vi "Setup for ISTR.vi"(7 "String":u8, 8 "error in (no error)":errorcluster, 9 "Position in":u32, 10 "Cree Comms in":refnum<class "Cree Communications.lvclass">, 11 "Calibration in":refnum<class "Calibration.lvclass">) -> (0 "error out":errorcluster, 1 "Position out":u32, 2 "Cree Comms out":refnum<class "Cree Communications.lvclass">, 3 "Calibration out":refnum<class "Calibration.lvclass">)   [LabVIEW 2015, in "Calibration.lvclass"]
doc: "Turns off the strings not being calibrated. Sets Dim command to 100."
uses:
  Calibration.lvclass
  Classes/Cree Communications/Class/Cree Communications.lvclass
  Classes/Cree Communications/Cree Comms Messages/Write Dim Level/Set Dim Level.lvclass
  Classes/Cree Communications/Cree Comms Messages/CC Message/CC Message.lvclass/CC Message.ctl
  Classes/Cree Communications/Cree Comms Messages/Set Current Reference/Set String Current Ref.lvclass
  Classes/Cree Communications/Cree Comms Messages/CC Message/CC Message.lvclass
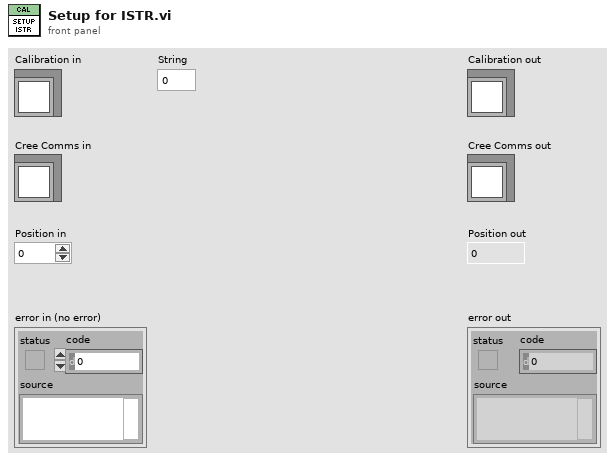
[diagram p1: front panel]
types:
  T1 = cluster{"Current Reference":dbl, "String":enum16{"Red", "BSY1", "BSY2"}}
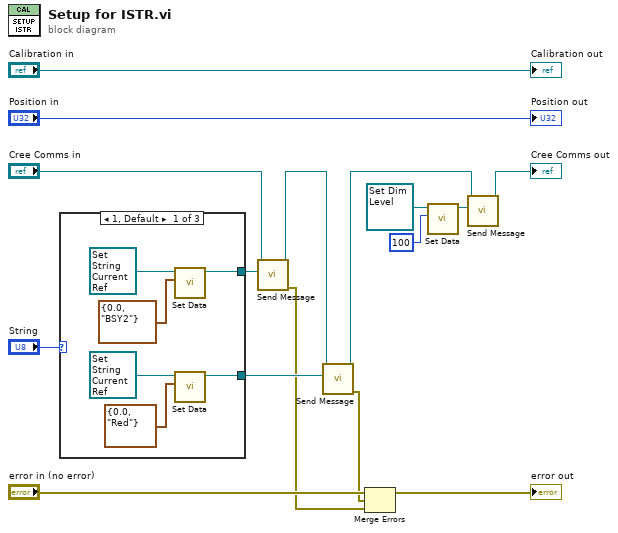
[diagram p0: block diagram]
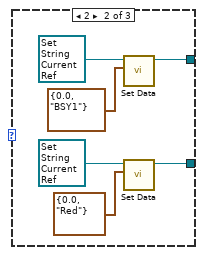
[diagram p2: hidden frame]
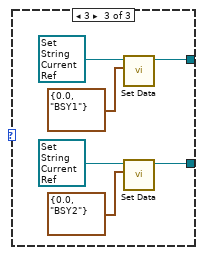
[diagram p3: hidden frame]
diagram:
  n1 = case shown="1, Default" "String" {
    tunnel: [w18 w24 w30] -> w10
    tunnel: [w17 w23 w29] -> w9
    frame 1, Default {
      n2 = call "Set Data.vi"("Data"=T1 {"Current Reference"=0.0, "String"=enum."BSY2"} ("Message Type"), "CC Message in"=refnum<class "Set String Current Ref.lvclass"> refnum ("Cree Comms Messages.lvlib:Set String Current Ref.lvclass")) -> ("CC Message out"=w18:refnum<class "Set String Current Ref.lvclass">)  [unwired: 8 in, 1 out]
      n3 = call "Set Data.vi"("Data"=T1 {"Current Reference"=0.0, "String"=enum."Red"} ("Message Type"), "CC Message in"=refnum<class "Set String Current Ref.lvclass"> refnum ("Cree Comms Messages.lvlib:Set String Current Ref.lvclass")) -> ("CC Message out"=w17:refnum<class "Set String Current Ref.lvclass">)  [unwired: 8 in, 1 out]
    }
    frame 2 {
      n4 = call "Set Data.vi"("Data"=T1 {"Current Reference"=0.0, "String"=enum."BSY1"} ("Message Type"), "CC Message in"=refnum<class "Set String Current Ref.lvclass"> refnum ("Cree Comms Messages.lvlib:Set String Current Ref.lvclass")) -> ("CC Message out"=w24:refnum<class "Set String Current Ref.lvclass">)  [unwired: 8 in, 1 out]
      n5 = call "Set Data.vi"("Data"=T1 {"Current Reference"=0.0, "String"=enum."Red"} ("Message Type"), "CC Message in"=refnum<class "Set String Current Ref.lvclass"> refnum ("Cree Comms Messages.lvlib:Set String Current Ref.lvclass")) -> ("CC Message out"=w23:refnum<class "Set String Current Ref.lvclass">)  [unwired: 8 in, 1 out]
    }
    frame 3 {
      n6 = call "Set Data.vi"("Data"=T1 {"Current Reference"=0.0, "String"=enum."BSY1"} ("Message Type"), "CC Message in"=refnum<class "Set String Current Ref.lvclass"> refnum ("Cree Comms Messages.lvlib:Set String Current Ref.lvclass")) -> ("CC Message out"=w30:refnum<class "Set String Current Ref.lvclass">)  [unwired: 8 in, 1 out]
      n7 = call "Set Data.vi"("Data"=T1 {"Current Reference"=0.0, "String"=enum."BSY2"} ("Message Type"), "CC Message in"=refnum<class "Set String Current Ref.lvclass"> refnum ("Cree Comms Messages.lvlib:Set String Current Ref.lvclass")) -> ("CC Message out"=w29:refnum<class "Set String Current Ref.lvclass">)  [unwired: 8 in, 1 out]
    }
  }
  n8 = call "Send Message.vi"("Cree Comms Message"=w10, "Acrobat Template in"="Cree Comms in") -> ("error out"=w6:errorcluster, "Acrobat Template out"=w11:refnum<class "Cree Communications.lvclass">)  [unwired: 8 in]
  n9 = call "Send Message.vi"("Cree Comms Message"=w9, "Acrobat Template in"=w11) -> ("error out"=w7:errorcluster, "Acrobat Template out"=w1:refnum<class "Cree Communications.lvclass">)  [unwired: 8 in]
  n10 = Merge Errors("error in (no error)", w7, w6) -> (→"error out":errorcluster)
  n11 = call "Set Data.vi"("Data"=u8 100 ("Message Type"), "CC Message in"=refnum<class "Set Dim Level.lvclass"> refnum ("Cree Comms Messages.lvlib:Set Dim Level.lvclass")) -> ("CC Message out"=w3:refnum<class "Set Dim Level.lvclass">)  [unwired: 8 in, 1 out]
  n12 = call "Send Message.vi"("Cree Comms Message"=w3, "Acrobat Template in"=w1) -> ("Acrobat Template out"=→"Cree Comms out":refnum<class "Cree Communications.lvclass">)  [unwired: 8 in, 1 out]
  "Calibration out" <- "Calibration in"
  "Position out" <- "Position in"
